vi "Basic Transmit and Receive.vi"() -> ()   [LabVIEW 2012, in "UART_Host_Driver.lvlib" / "UART Driver.lvclass"]
doc: "This example calls the UART Initialize, UART Configure Port, UART Execute Command, and a UART Close."
uses:
  UART Driver.lvclass
  Typedefs/Configuration Parameters.ctl
  FPGA/UART/StopBits.ctl
  FPGA/UART/Parity.ctl
  FPGA/UART/UART_Firmware.lvlib
  UART_Host_Driver.lvlib
panel:
  in  "Rx byte count":u32=4
  in  "Configuration Parameters":T1={"Baud"=115200, "Character Length"=8, "Stop Bits"=enum."1.0", "Parity"=enum."None", "Character Spacing (ticks)"=0}
  out "Receive Data":string
  in  "Tx Data":string="TEST"
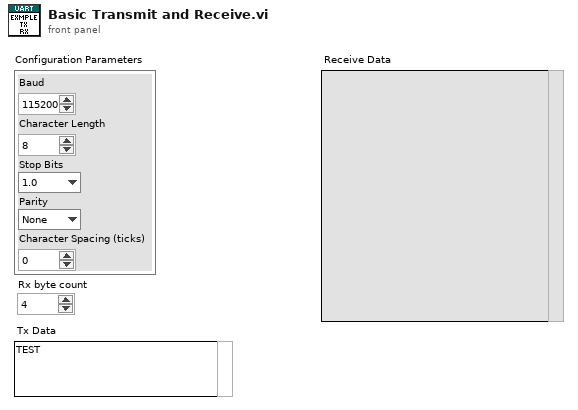
[diagram p1: front panel]
types:
  T1 = typedef "UART_Host_Driver.lvlib/Configuration Parameters.ctl" = cluster{"Baud":u32, "Character Length":u8, "Stop Bits":T2, "Parity":T3, "Character Spacing (ticks)":u32}
  T2 = typedef "UART_Firmware.lvlib/StopBits.ctl" = enum8{"1.0", "1.5", "2.0"}
  T3 = typedef "UART_Firmware.lvlib/Parity.ctl" = enum8{"None", "Even", "Odd"}
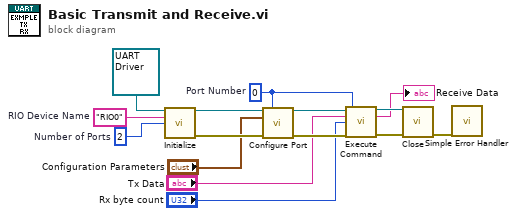
[diagram p0: block diagram]
diagram:
  w4 = u8 0  # Port Number
  w9 = u8 2  # Number of Ports
  w10 = "RIO0"  # RIO Device Name
  n1 = call-dynamic "Initialize.vi"("UART Driver in"=refnum<class "UART Driver.lvclass"> refnum, "RIO Device Name"=w10, "Number of UART Controllers"=w9) -> ("UART Driver out"=w15:refnum<class "UART Driver.lvclass">, "error out"=w14:errorcluster)  [unwired: 11 in]
  n2 = call-dynamic "Configure Port.vi"("UART Driver in"=w15, "Controller Number"=w4, "Configuration Parameters"="Configuration Parameters", "error in"=w14) -> ("UART Driver out"=w13:refnum<class "UART Driver.lvclass">, "error out"=w12:errorcluster)  [unwired: 10 in]
  n3 = call-dynamic "Execute Command.vi"("UART Driver in"=w13, "Port Number"=w4, "Tx Data"="Tx Data", "Rx byte count"="Rx byte count", "error in"=w12) -> ("UART Driver out"=w8:refnum<class "UART Driver.lvclass">, "Receive Data"=→"Receive Data":string, "error out"=w7:errorcluster)  [unwired: 8 in]
  n4 = call-dynamic "Close.vi"("UART Driver in"=w8, "error in"=w7) -> ("error out"=w6:errorcluster)  [unwired: 13 in]
  n5 = call <vilib>:"Simple Error Handler.vi"("error in (no error)"=w6) -> ()  [unwired: 4 in, 5 out]
